vi "comhpuertas logicas.vi"() -> ()   [LabVIEW 2013]
panel:
  out "Boolean 6":bool
  in  "Boolean 5":bool
  in  "Boolean 4":bool
  out "Boolean 3":bool
  in  "Boolean 2":bool
  in  "Boolean":bool
  out "G=Z+W":bool
  in  "W":bool
  in  "?":bool
  out "F=XY":bool
  in  "Y":bool
  in  "X":bool
  # "Z"
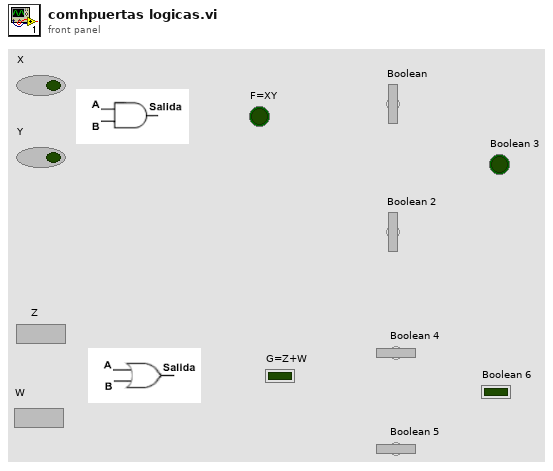
[diagram p1: front panel]
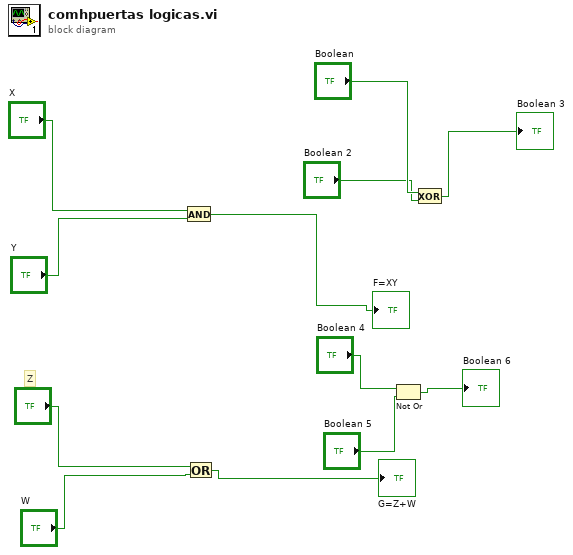
[diagram p0: block diagram]
diagram:
  # "Z"
  n1 = And(x="X", y="Y") -> (x .and. y?=→"F=XY":bool)
  n2 = Or(x="?", y="W") -> (x .or. y?=→"G=Z+W":bool)
  n3 = Not Or(1:"Boolean 5", 2:"Boolean 4") -> (0:→"Boolean 6":bool)
  n4 = Exclusive Or(1:"Boolean 2", 2:"Boolean") -> (0:→"Boolean 3":bool)
